vi "soundGenerator.vi"(9 "Start":bool, 10 "Duration (s)":dbl, 11 "Frequency":dbl(knob) scale=0.0..5000.0) -> (3 "Countdown":dbl)   [LabVIEW 2009]
uses:
  <vilib>/measure/NI_MABase.lvlib
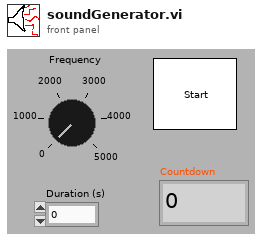
[diagram p1: front panel]
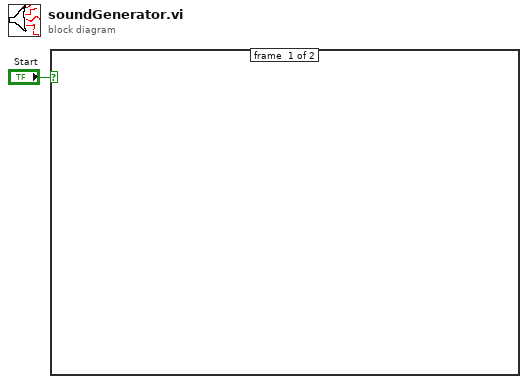
[diagram p0: block diagram]
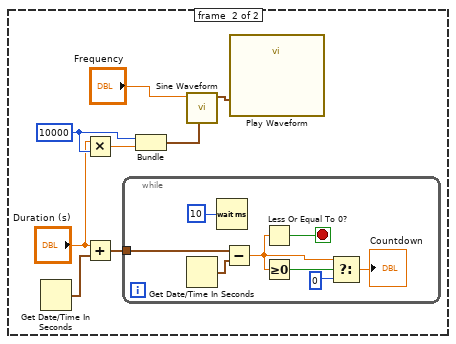
[diagram p2: hidden frame]
diagram:
  n1 = case shown="True" "Start" {
    frame #0 {
    }
    frame #1 {
      w5 = 10000
      n2 = Get Date/Time In Seconds() -> (seconds since 1Jan1904=w3:timestamp)
      n3 = Multiply(x="Duration (s)", y=w5) -> (x*y=w6:dbl)
      n4 = Add(x="Duration (s)", y=w3) -> (x+y=w2:timestamp)
      n5 = while {
        tunnel: w2 -> [w17]
        stop <- w13 stop-if-true
        n6 = Get Date/Time In Seconds() -> (seconds since 1Jan1904=w16:timestamp)
        n7 = Wait (ms)(milliseconds to wait=u32 10) -> ()  [unwired: 1 out]
        n8 = Subtract(x=w17, y=w16) -> (x-y=w11:dbl)
        n9 = Less Or Equal To 0?(x=w11) -> (x <= 0?=w13:bool)
        n10 = Greater Or Equal To 0?(x=w11) -> (x >= 0?=w10:bool)
        n11 = Select(t=w11, s=w10, f=0) -> (s? t:f=→"Countdown":dbl)
      }
      n12 = Bundle(w5, w6) -> (w7:cluster{i32, dbl})  [unwired: 1 in]
      n13 = call <vilib>:"Sine Waveform.vi"("sampling info"=w7, "frequency"="Frequency") -> ("signal out"=w8:waveform(dbl))  [unwired: 8 in, 1 out]
      n14 = call "Play Waveform"("Data"=w8) -> ()  [unwired: 18 in, 1 out]
    }
  }
